vi "Configure Averaging.vi"(0 "VISA resource name":refnum<visa-resource-name>, 1 "Enable Average Duration (F: Disable)":bool, 2 "Enable Averaging (F: Disable)":bool, 5 "Trace (1: Trace 1)":i32(ring)=1 items=["Trace 1"=1, "Trace 2"=2, "Trace 3"=3, "Trace 4"=4], 7 "Averaging Duration (0)":dbl, 9 "Average Count (100)":i32=100, 11 "error in (no error)":errorcluster, 12 "Averaging Type (0: Log Power)":i32(ring) items=["Log Power", "Power", "Voltage"]) -> (4 "VISA resource name out":refnum<visa-resource-name>, 15 "error out":errorcluster)   [LabVIEW 2022 SP3, in "Agilent N934X Series.lvlib"]
doc: "Configures the averaging."
uses:
  <instrlib>/Agilent N934X Series/Agilent N934X Series.lvlib
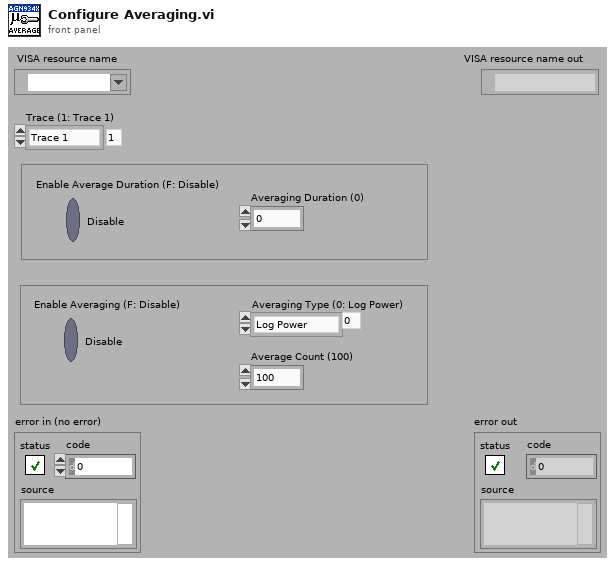
[diagram p1: front panel]
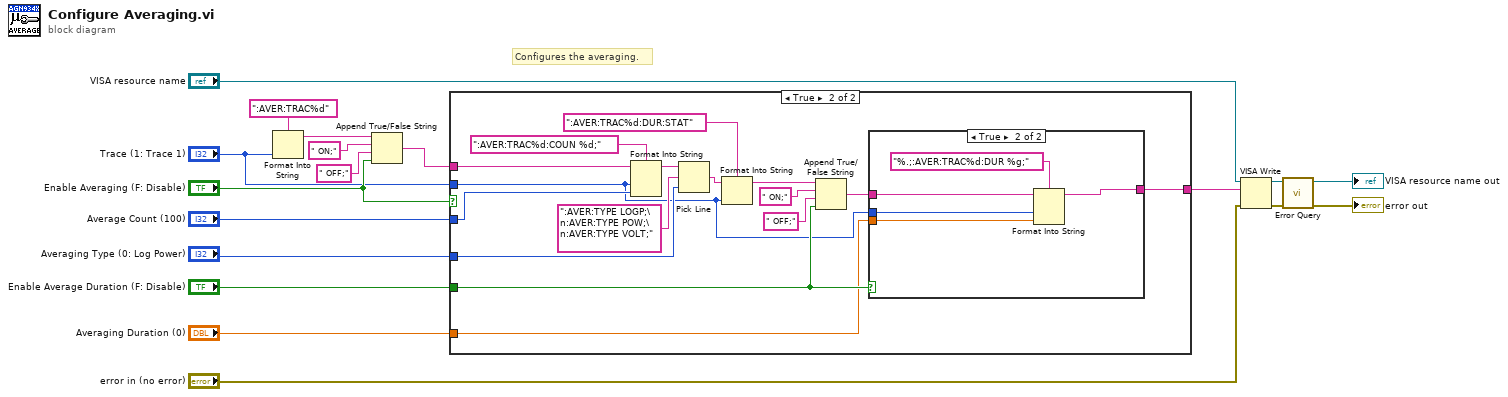
[diagram p0: block diagram]
diagram:
  # "Configures the averaging."
  n1 = Format Into String(format string=":AVER:TRAC%d", "Trace (1: Trace 1)") -> (resulting string=w10:string)  [unwired: 2 in, 1 out]
  n2 = Append True/False String(1:"Enable Averaging (F: Disable)", 2:" OFF;" ("false string"), 3:" ON;" ("false string"), 4:w10) -> (0:w6:string)
  n3 = case shown="True" "Enable Averaging (F: Disable)" {
    tunnel: "Trace (1: Trace 1)" -> [_ w23]
    tunnel: "Average Count (100)" -> [_ w34]
    tunnel: w6 -> [w19 w33]
    tunnel: "Averaging Type (0: Log Power)" -> [_ w30]
    tunnel: "Enable Average Duration (F: Disable)" -> [_ w25]
    tunnel: "Averaging Duration (0)" -> [_ w22]
    tunnel: [w19 w21] -> w3
    frame False {
    }
    frame True {
      n4 = Format Into String(format string=":AVER:TRAC%d:COUN %d;", initial string=w33, w23, w34) -> (resulting string=w31:string)  [unwired: 1 in, 1 out]
      n5 = Pick Line(string ("")=w31, multi-line string=":AVER:TYPE LOGP;\n:AVER:TYPE POW;\n:AVER:TYPE VOLT;", line index=w30) -> (output string=w29:string)
      n6 = Format Into String(format string=":AVER:TRAC%d:DUR:STAT", initial string=w29, w23) -> (resulting string=w26:string)  [unwired: 1 in, 1 out]
      n7 = Append True/False String(1:w25, 2:" OFF;" ("false string"), 3:" ON;" ("false string"), 4:w26) -> (0:w24:string)
      n8 = case shown="True" w25 {
        tunnel: w24 -> [w36 w41]
        tunnel: w23 -> [_ w40]
        tunnel: w22 -> [_ w39]
        tunnel: [w36 w38] -> w21
        frame False {
        }
        frame True {
          n9 = Format Into String(format string="%.;:AVER:TRAC%d:DUR %g;", initial string=w41, w40, w39) -> (resulting string=w38:string)  [unwired: 1 in, 1 out]
        }
      }
    }
  }
  n10 = VISA Write(VISA resource name="VISA resource name", write buffer=w3, error in (no error)="error in (no error)") -> (VISA resource name out=w16:refnum<visa-resource-name>, error out=w15:errorcluster)  [unwired: 1 out]
  n11 = call <instrlib>:"Error Query.vi"("error in (no error)"=w15, "VISA resource name"=w16) -> ("error out"=→"error out":errorcluster, "VISA resource name out"=→"VISA resource name out":refnum<visa-resource-name>)  [unwired: 6 in, 2 out]
